vi "校准_开始消息.vi"(9 "COM":i32, 10 "A":i32) -> ()   [LabVIEW 2015]
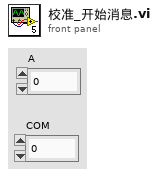
[diagram p1: front panel]
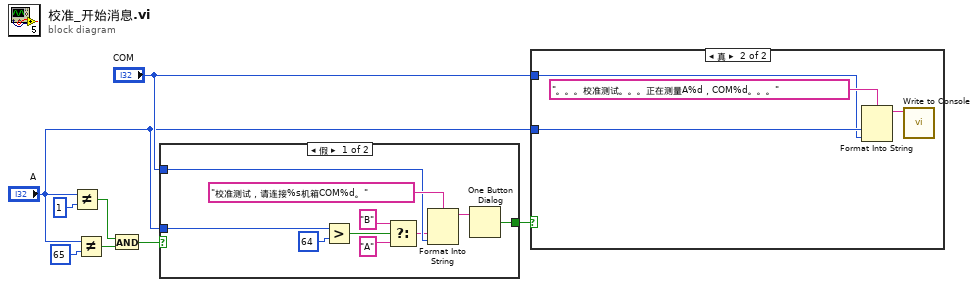
[diagram p0: block diagram]
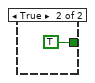
[diagram p2: hidden frame]
diagram:
  n1 = Not Equal?(x="A", y=1) -> (x != y?=w3:bool)
  n2 = Not Equal?(x="A", y=65) -> (x != y?=w2:bool)
  n3 = And(x=w3, y=w2) -> (x .and. y?=w1:bool)
  n4 = case shown="假" w1 {
    tunnel: [w18 TRUE ("true")] -> w8
    tunnel: "COM" -> [w14 _]
    tunnel: "A" -> [w9 _]
    frame False {
      n5 = Greater?(x=w9, y=64) -> (0:w13:bool)
      n6 = Select(t="B" ("format string"), s=w13, f="A" ("format string")) -> (s? t:f=w10:string)
      n7 = Format Into String(format string="校准测试，请连接%s机箱COM%d。", w10, w14) -> (resulting string=w17:string)  [unwired: 2 in, 1 out]
      n8 = One Button Dialog(message=w17) -> (true=w18:bool)  [unwired: 1 in]
    }
    frame True {
    }
  }
  n9 = case shown="真" w8 {
    tunnel: "A" -> [_ w22]
    tunnel: "COM" -> [_ w21]
    frame False {
    }
    frame True {
      n10 = Format Into String(format string="。。。校准测试。。。正在测量A%d，COM%d。。。", w22, w21) -> (resulting string=w20:string)  [unwired: 2 in, 1 out]
      n11 = call "Write to Console.vi"("Input"=w20) -> ()  [unwired: 10 in, 1 out]
    }
  }
